vi "MongoDB.ConnectionOpen.vi"(8 "error in (no error)":errorcluster, 10 "connectionString":string) -> (0 "error out":errorcluster, 3 "MongoDB out":refnum<class "MongoDB.Client.lvclass">)   [LabVIEW 2014, in "MongoDB.Client.lvclass"]
uses:
  MongoDB.Client.lvclass
  C:/Users/Richard/Documents/GitHub/mongo-labview-driver/CSharp/bin/MongoDB.Driver.Legacy.dll
  CSharp/bin/MongoDB.Driver.Legacy.dll
  C:/Users/Richard/Documents/GitHub/mongo-labview-driver/CSharp/bin/MongoDB.Driver.dll
  CSharp/bin/MongoDB.Driver.dll
  MongoDB.Client.lvclass/MongoDB.Client.ctl
panel:
  in  "MongoClientExtensions":refnum<k24>
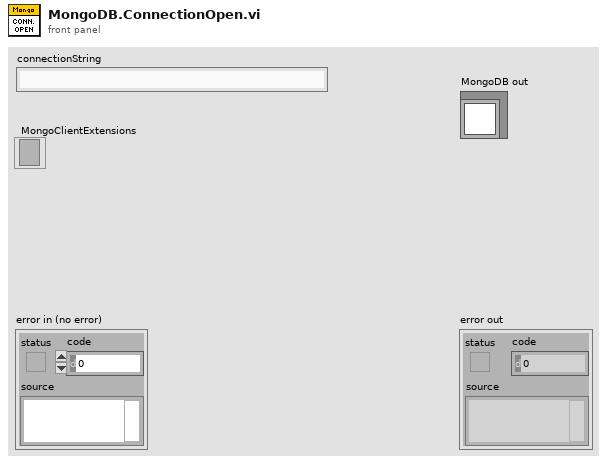
[diagram p1: front panel]
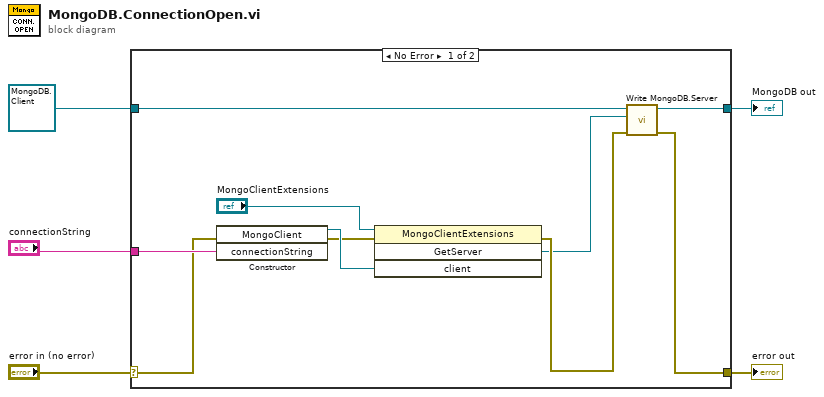
[diagram p0: block diagram]
diagram:
  n1 = case shown="No Error" "error in (no error)" {
    selector: "error in (no error)" -> [w11 w17]
    tunnel: [w8 w17] -> w4
    tunnel: [w10 w16] -> w3
    tunnel: "connectionString" -> [w12 _]
    tunnel: refnum<class "MongoDB.Client.lvclass"> refnum ("MongoDB.Client in") -> [w6 w16]
    frame No Error {
      n2 = constructor class="MongoClient"(error in=w11, "connectionString"=w12) -> (reference out=w14:refnum<k24>, error out=w13:errorcluster)  [unwired: 2 in, 2 out]
      n3 = invoke class="MongoClientExtensions" method="GetServer"(reference="MongoClientExtensions", error in=w13, "client"=w14) -> (error out=w9:errorcluster, "GetServer"=w7:refnum<k24>)  [unwired: 1 in, 2 out]
      n4 = call "Write MongoDB.Server.vi"("error in (no error)"=w9, "MongoDB.Server"=w7, "MongoDB.Client in"=w6) -> ("error out"=w8:errorcluster, "MongoDB.Client out"=w10:refnum<class "MongoDB.Client.lvclass">)  [unwired: 7 in]
    }
    frame Error {
    }
  }
  "error out" <- w4
  "MongoDB out" <- w3
